vi "outputCluster-to-dbColumnInfo.vi"(4 "cluster ref":refnum<vi>) -> (7 "Column Information":T1[](array[typedef]))   [LabVIEW 2011]
uses:
  <vilib>/addons/database/Auxilliary.llb/DB Tools Column Info.ctl
  <vilib>/addons/database/Auxilliary.llb/DB Tools DataTypes.ctl
  <vilib>/addons/database/NI_Database_API.lvlib
panel:
  out "Label.Text":string
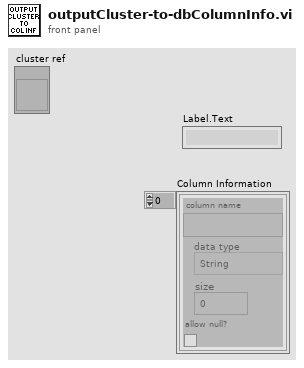
[diagram p1: front panel]
types:
  T1 = typedef "NI_Database_API.lvlib/DB Tools Column Info.ctl" = cluster{"column name":string, "data type":T2, "size":i32, "allow null?":bool}
  T2 = typedef "NI_Database_API.lvlib/DB Tools DataTypes.ctl" = enum16{"String", "Long (I32)", "Single (SGL)", "Double (DBL)", "Date/Time", "Binary"}
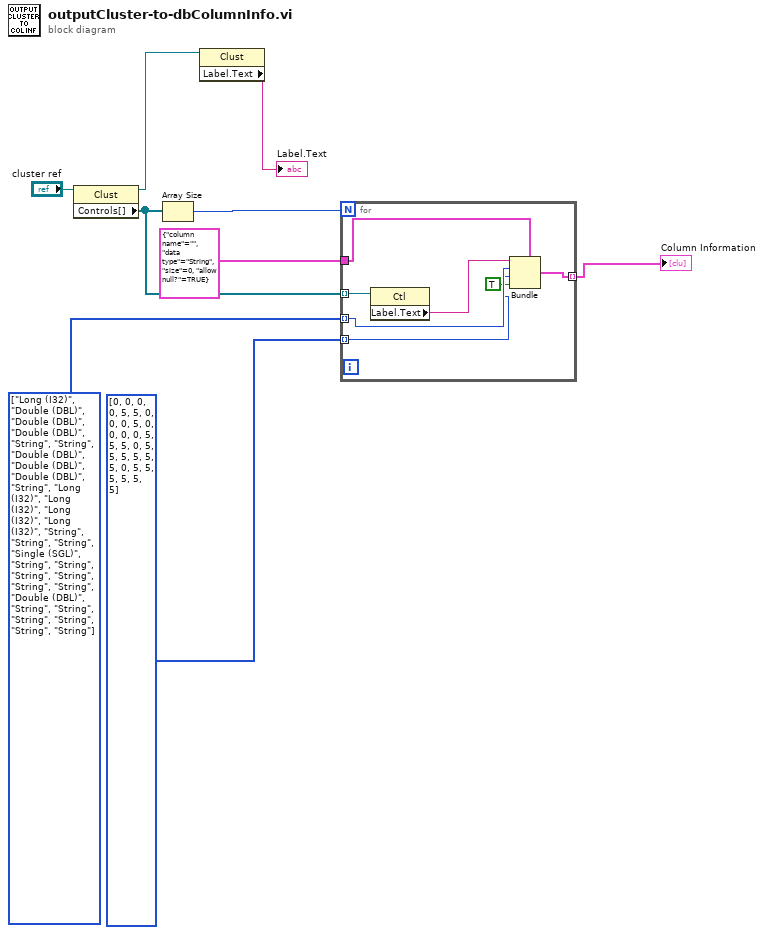
[diagram p0: block diagram]
diagram:
  w2 = T2[] [enum."Long (I32)", enum."Double (DBL)", enum."Double (DBL)", enum."Double (DBL)", enum."String", enum."String", enum."Double (DBL)", enum."Double (DBL)", enum."Double (DBL)", enum."String", enum."Long (I32)", enum."Long (I32)", enum."Long (I32)", enum."Long (I32)", enum."String", enum."String", enum."String", enum."Single (SGL)", enum."String", enum."String", enum."String", enum."String", enum."String", enum."String", enum."Double (DBL)", enum."String", enum."String", enum."String", enum."String", enum."String", enum."String"] items=["String", "Long (I32)", "Single (SGL)", "Double (DBL)", "Date/Time", "Binary"]
  n1 = property class="Clust"(reference="cluster ref") -> (reference out=w9:refnum<vi>, "Controls[]"=w7:refnum<vi>[])  [unwired: 1 in, 1 out]
  n2 = Array Size(array=w7) -> (size(s)=w6:i32)
  n3 = property class="Clust"(reference=w9) -> ("Label.Text"=→"Label.Text":string)  [unwired: 1 in, 2 out]
  n4 = for {
    N: w6 -> [_]
    tunnel: w7 -> [w16] mode=indexing
    tunnel: [w13] -> w3 mode=indexing
    tunnel: T1 {"column name"="", "data type"=enum."String", "size"=0, "allow null?"=TRUE} ("column information") -> [w15]
    tunnel: w2 -> [w12] mode=indexing
    tunnel: i32[] [0, 0, 0, 0, 5, 5, 0, 0, 0, 5, 0, 0, 0, 0, 5, 5, 5, 0, 5, 5, 5, 5, 5, 5, 0, 5, 5, 5, 5, 5, 5] -> [w11] mode=indexing
    n5 = property class="Ctl"(reference=w16) -> ("Label.Text"=w14:string)  [unwired: 1 in, 2 out]
    n6 = Bundle(cluster=w15, "column name"=w14, "data type"=w12, "size"=w11, "allow null?"=TRUE) -> (w13:T1)
  }
  "Column Information" <- w3
